vi "Depth of Tree.vi"(11 "Tree in":T1) -> (2 "Depth":i32, 3 "Tree with Depths":T1)   [LabVIEW 2025]
uses:
  Types/Decision Tree.ctl
  Types/Sequencing Tree Node.ctl
  Types/Single Cmd Info.ctl
  <vilib>/picture/picture.llb/imagedata.ctl
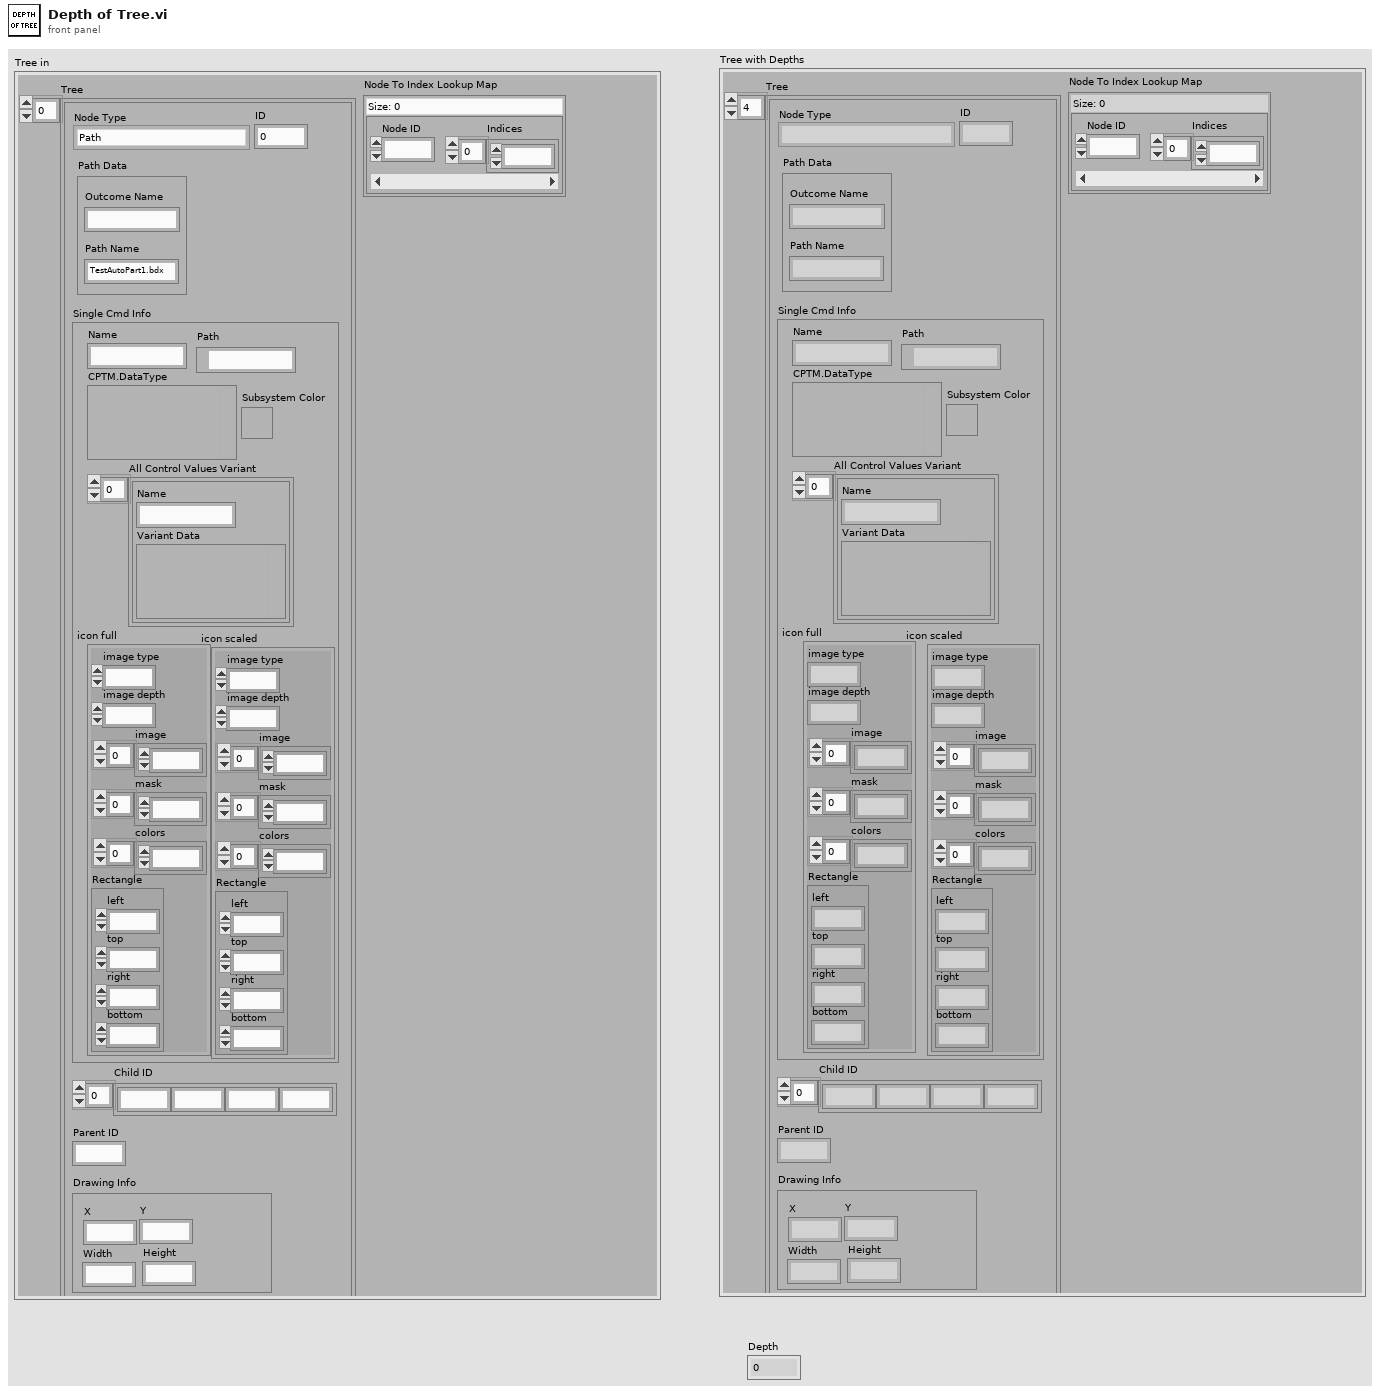
[diagram p1: front panel]
types:
  T1 = typedef "Decision Tree.ctl" = cluster{"Tree":T2[], "Node To Index Lookup Map":map{i16, i16[]}}
  T2 = typedef "Sequencing Tree Node.ctl" = cluster{"Node Type":enum16{"Path", "Command", "Leaf"}, "ID":i16, "Path Data":cluster{"Path Name":string, "Outcome Name":string}, "Single Cmd Info":T3, "Child ID":i32[], "Parent ID":i32, "Drawing Info":cluster{"X":i32, "Y":i32, "Width":i32, "Height":i32}}
  T3 = typedef "Single Cmd Info.ctl" = cluster{"Name":string, "CPTM.DataType":variant, "All Control Values Variant":cluster{"Name":string, "Variant Data":variant}[], "icon full":T4, "icon scaled":T4, "Path":path, "Subsystem Color":u32}
  T4 = typedef "imagedata.ctl" = cluster{"image type":i32, "image depth":i32, "image":u8[], "mask":u8[], "colors":u32[], "Rectangle":cluster{"left":i16, "top":i16, "right":i16, "bottom":i16}}
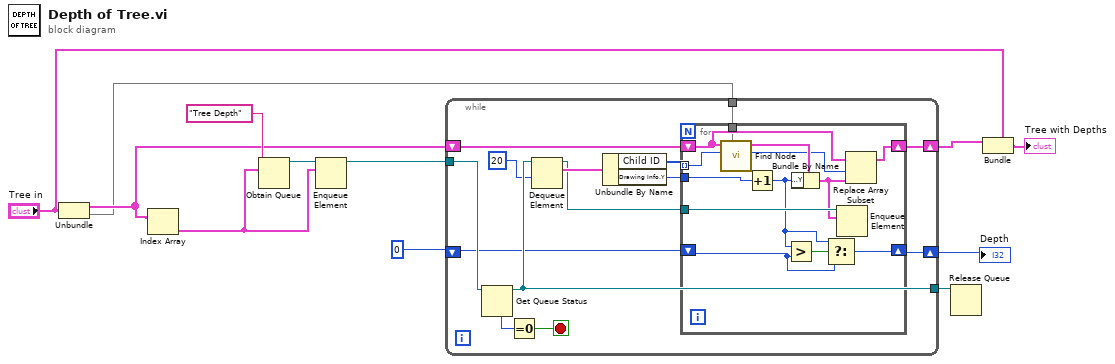
[diagram p0: block diagram]
diagram:
  n1 = Unbundle("Tree in") -> ("Tree"=w5:T2[], "Node To Index Lookup Map"=w2:map{i16, i16[]})
  n2 = Index Array(array=w5) -> (element=w6:T2)  [unwired: 1 in]
  n3 = Obtain Queue(name (unnamed)="Tree Depth", element data type=w6) -> (queue out=w8:refnum<queue>)  [unwired: 3 in, 2 out]
  n4 = Enqueue Element(queue=w8, element=w6) -> (queue out=w9:refnum<queue>)  [unwired: 2 in, 2 out]
  n5 = while {
    tunnel: w9 -> [w20]
    shift-right: [w22] -> w4
    shift-left: w5 -> [w23]
    tunnel: [w18] -> w10
    shift-right: [w14] -> w12
    shift-left: 0 -> [w15]
    tunnel: w2 -> [w13]
    stop <- w26 stop-if-true
    n6 = Get Queue Status(queue=w20) -> (queue out=w18:refnum<queue>, # elements in queue=w21:i32)  [unwired: 2 in, 6 out]
    n7 = Equal To 0?(x=w21) -> (x = 0?=w26:bool)
    n8 = Dequeue Element(queue=w18, timeout in ms (-1)=20) -> (queue out=w19:refnum<queue>, element=w25:T2)  [unwired: 1 in, 2 out]
    n9 = Unbundle By Name(w25) -> ("Child ID"=w24:i32[], "Drawing Info.Y"=w16:i32)
    n10 = for {
      tunnel: w24 -> [w29] mode=indexing
      tunnel: w16 -> [w39]
      shift-right: [w37] -> w22
      shift-left: w23 -> [w30]
      tunnel: w19 -> [w36]
      shift-right: [w31] -> w14
      shift-left: w15 -> [w32]
      tunnel: w13 -> [w27]
      n11 = call "Find Node.vi"("Node To Index Lookup Map"=w27, "ID"=w29, "Tree"=w30) -> ("Index"=w28:i16, "Node"=w38:T2)  [unwired: 7 in]
      n12 = Increment(x=w39) -> (x+1=w33:i32)
      n13 = Greater?(x=w33, y=w32) -> (0:w34:bool)
      n14 = Bundle By Name(cluster=w38, "Drawing Info.Y"=w33) -> (w35:T2)
      n15 = Select(t=w33, s=w34, f=w32) -> (s? t:f=w31:i32)
      n16 = Enqueue Element(queue=w36, element=w35) -> ()  [unwired: 2 in, 3 out]
      n17 = Replace Array Subset(array=w30, new element=w35, index=w28) -> (w37:T2[])
    }
  }
  "Depth" <- w12
  n18 = Release Queue(queue=w10) -> ()  [unwired: 2 in, 3 out]
  n19 = Bundle(cluster="Tree in", "Tree"=w4) -> (→"Tree with Depths":T1)  [unwired: 1 in]
